vi "GetCtlRef_Core.vi"(8 "error in (no error)":errorcluster, 10 "CtlName In":string, 11 "ctlrRef_VAT in":refnum<class "ctlRef_VAT.lvclass">) -> (0 "error out":errorcluster, 1 "Ctl Refnum":refnum<vi>, 2 "CtlName out":string, 3 "ctlrRef_VAT out":refnum<class "ctlRef_VAT.lvclass">, 4 "Found":bool)   [LabVIEW 2020, in "CtlReferences.lvlib" / "ctlRef_VAT.lvclass"]
uses:
  ctlRef_VAT.lvclass
  ctlRef_VAT.lvclass/ctlRef_VAT.ctl
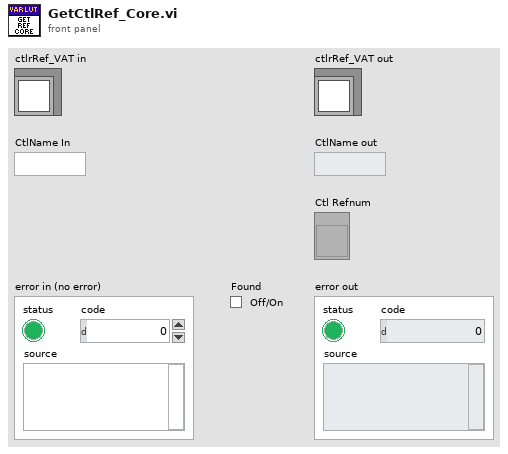
[diagram p1: front panel]
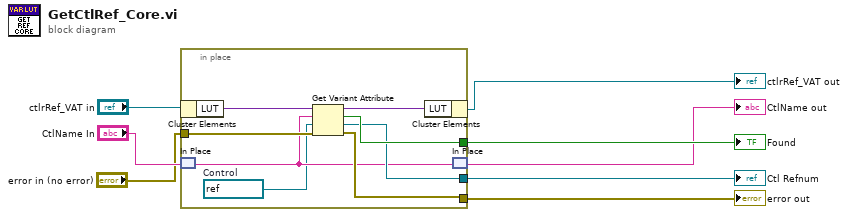
[diagram p0: block diagram]
diagram:
  n1 = in-place {
    in-place-border: "error in (no error)" -> [w16]
    in-place-border: [w15] -> w4
    in-place-border: [w14] -> w5
    in-place-border: [w11] -> w3
    w9 = refnum<vi> refnum  # Control
    n2 = in-place-cluster #1("ctlrRef_VAT in") -> ("LUT"=w13:variant)
    n3 = in-place-match #2("CtlName In") -> (w10:string)
    n4 = Get Variant Attribute(Variant=w13, name=w10, default value (empty Variant)=w9, error in=w16) -> (duplicate Variant=w12:variant, found=w15:bool, value=w11:refnum<vi>, error out=w14:errorcluster)
    n5 = in-place-cluster #1("LUT"=w12) -> (→"ctlrRef_VAT out":refnum<class "ctlRef_VAT.lvclass">)
    n6 = in-place-match #2(w10) -> (→"CtlName out":string)
  }
  "Ctl Refnum" <- w3
  "error out" <- w5
  "Found" <- w4
